vi "GetSingleIncomingCh.vi"(0 "Device Ref in":T1 format="%.0x", 3 "error in (no error)":errorcluster) -> (7 "Device Ref out":T1 format="%.0x", 8 "Channel Data Ref":T2[](array[typedef]) format="%.0x", 9 "FR Signals":refnum<k21>[](array[refnum]), 10 "error out":errorcluster)   [LabVIEW 2020, in "FlexRay Custom Device Engine.lvlib"]
uses:
  FlexRay Custom Device Engine.lvlib
  <vilib>/NI VeriStand/Custom Device API/Custom Device Item Ref.ctl
  <vilib>/NI VeriStand/Custom Device API/Data Reference.ctl
  <vilib>/NI VeriStand/Custom Device API/Data Access Type.ctl
  <vilib>/NI VeriStand/Custom Device API/Custom Device API.lvlib
  <vilib>/NI VeriStand/Custom Device Tools/Custom Device Utility Library/Custom Device Utility Library.lvlib
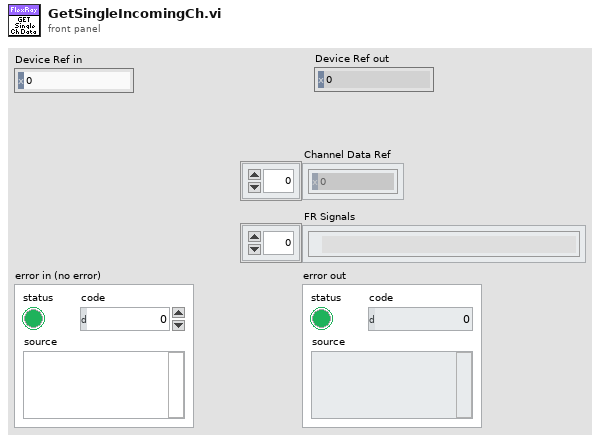
[diagram p1: front panel]
types:
  T1 = typedef "Custom Device API.lvlib/Custom Device Item Ref.ctl" = u64
  T2 = typedef "Custom Device API.lvlib/Data Reference.ctl" = i32
  T3 = typedef "Custom Device API.lvlib/Data Access Type.ctl" = enum16{"Read", "Write"}
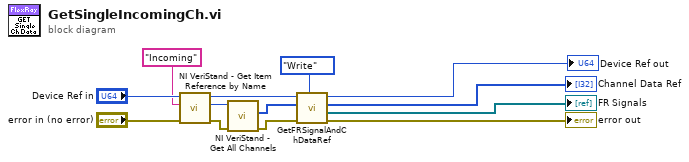
[diagram p0: block diagram]
diagram:
  n1 = call <vilib>:"NI VeriStand - Get Item Reference by Name.vi"("error in (no error)"="error in (no error)", "Item Name"="Incoming" ("Section Name"), "Parent Ref in"="Device Ref in") -> ("error out"=w4:errorcluster, "Item Ref"=w3:T1, "Parent Ref out"=w5:T1)  [unwired: 5 in, 1 out]
  n2 = call <vilib>:"NI VeriStand - Get All Channels.vi"("error in"=w4, "Section Ref in"=w3) -> ("error out"=w6:errorcluster, "Channel Refs"=w7:T1[])  [unwired: 6 in, 2 out]
  n3 = call "GetFRSignalAndChDataRef.vi"("Access"=Data_Access_Type."Write", "error in (no error)"=w6, "Channel Refs"=w7, "Device Ref in"=w5) -> ("error out"=→"error out":errorcluster, "FR Signals"=→"FR Signals":refnum<k21>[], "Channel Data Ref"=→"Channel Data Ref":T2[], "Device Ref out"=→"Device Ref out":T1)  [unwired: 4 in]
